vi "Logging Message Loop.vi"(8 "error in (no error)":cluster{"状态":bool, "代码":i32, "源":string} caption="错误输入（无错误）", 10 "数据队列":refnum<queue>, 11 "消息队列":T1) -> (0 "error out":cluster{"状态":bool, "代码":i32, "源":string} caption="错误输出")   [LabVIEW 2015, in "DAQ.lvlib"]
doc: "消息循环子VI负责处理与记录数据相关的消息。"
uses:
  DAQ.lvlib
  support/Message Queue/All Message Queues Sample Panel.ctl
  support/Message Queue/Message Cluster.ctl
  Support/Logging Configuration.ctl
  Support/Logging State.ctl
  support/Message Queue/Enqueue Message (Single).vi
  <vilib>/Utility/error.llb/Error Cluster From Error Code.vi
  <vilib>/ErrorRing/Error Ring.xnode
  support/Message Queue/Message Queue.lvlib
  Utility VIs/Utility VIs.lvlib
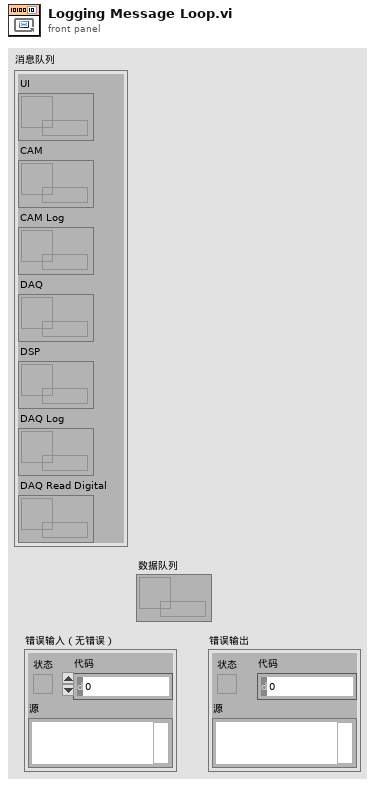
[diagram p1: front panel]
types:
  T1 = typedef "Message Queue.lvlib/All Message Queues Sample Panel.ctl" = cluster{"UI":refnum<queue>, "CAM":refnum<queue>, "CAM Log":refnum<queue>, "DAQ":refnum<queue>, "DSP":refnum<queue>, "DAQ Log":refnum<queue>, "DAQ Read Digital":refnum<queue>}
  T2 = typedef "DAQ.lvlib/Logging State.ctl" = enum16{"Idle", "Logging"}
  T3 = typedef "DAQ.lvlib/Logging Configuration.ctl" = cluster{"记录文件基路径":path}
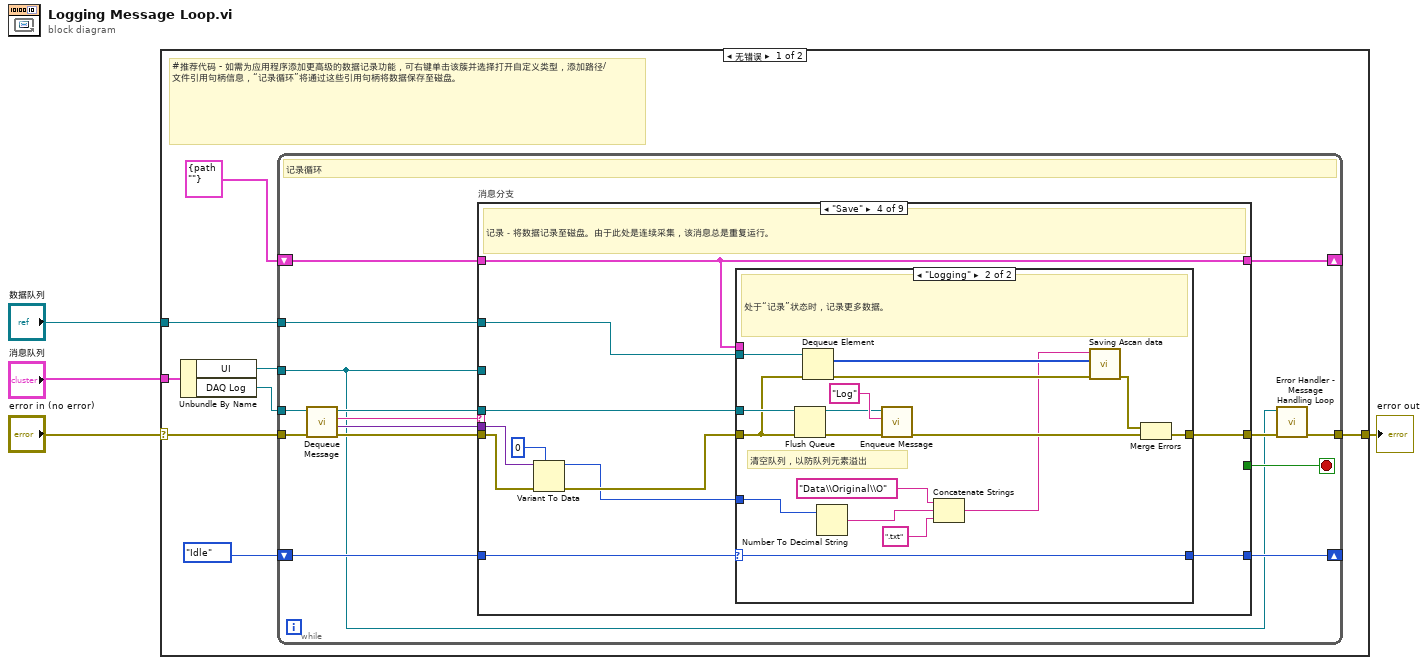
[diagram p0: block diagram]
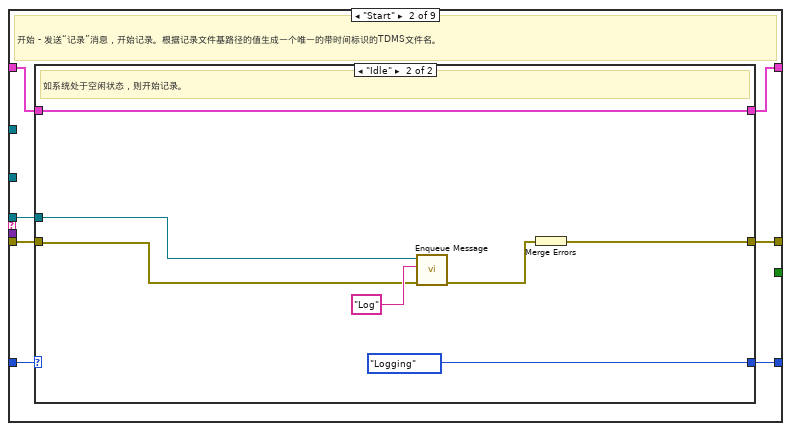
[diagram p3: hidden frame]
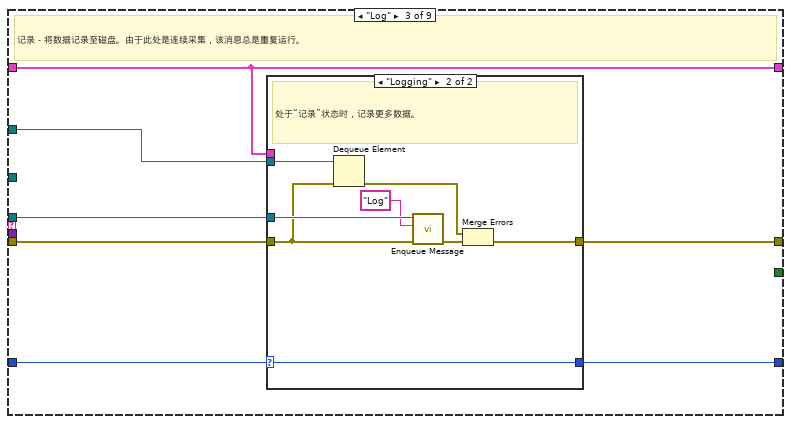
[diagram p5: hidden frame]
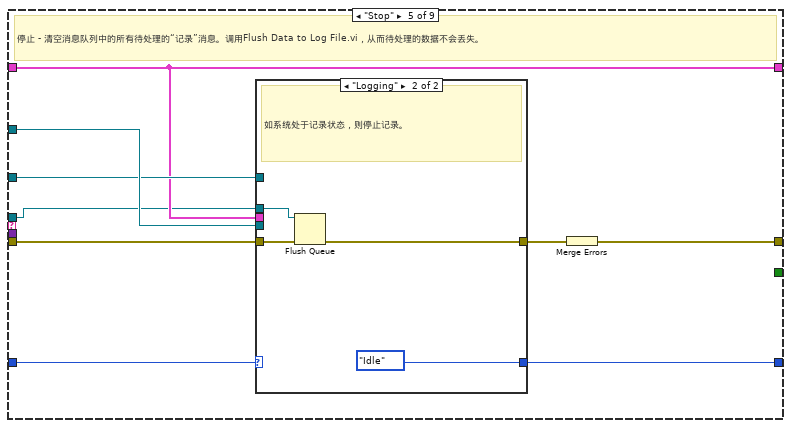
[diagram p8: hidden frame]
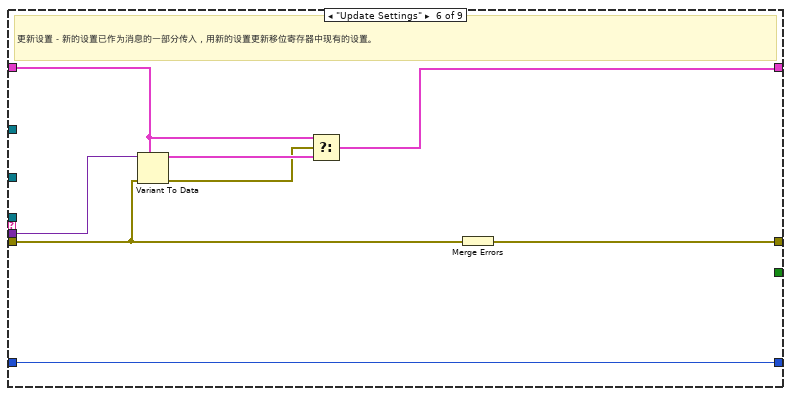
[diagram p10: hidden frame]
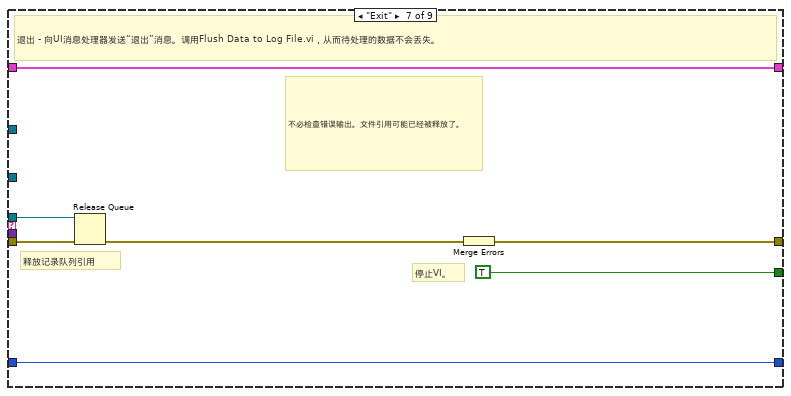
[diagram p11: hidden frame]
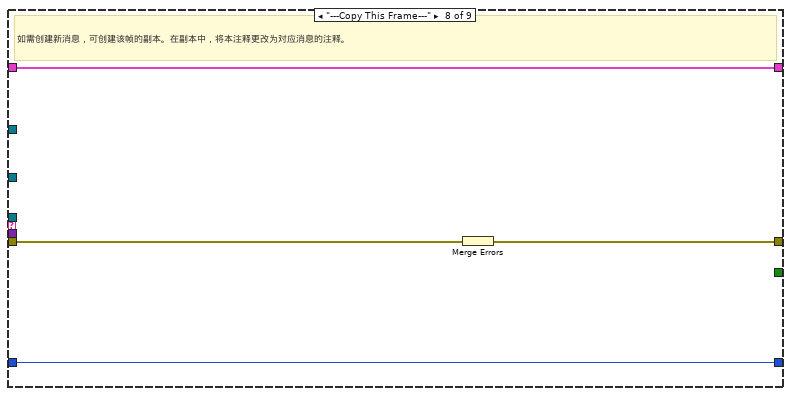
[diagram p12: hidden frame]
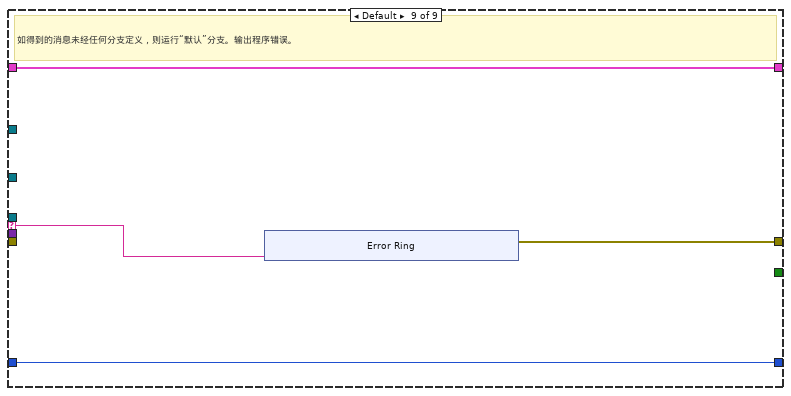
[diagram p13: hidden frame]
diagram:
  n1 = case shown="无错误" "error in (no error)" {
    selector: "error in (no error)" -> [w9 w140]
    tunnel: "消息队列" -> [w12 _]
    tunnel: [w10 w140] -> w4
    tunnel: "数据队列" -> [w8 _]
    frame No Error {
      # "#推荐代码 - 如需为应用程序添加更高级的数据记录功能，可右键单击该簇并选择打开自定义类型，添加路径/文件引用句柄信息，“记录循环”将通过这些引用句柄将数据保存至磁盘。"
      n2 = Unbundle By Name(w12) -> ("UI"=w7:refnum<queue>, "DAQ Log"=w11:refnum<queue>)
      n3 = while {
        tunnel: w11 -> [w19]
        shift-right: [w26] -> _
        shift-left: T3 {"记录文件基路径"=path ""} ("记录配置") -> [w27]
        tunnel: w7 -> [w13]
        tunnel: w8 -> [w18]
        shift-right: [w16] -> _
        shift-left: Logging_State."Idle" ("记录状态") -> [w17]
        tunnel: w9 -> [w24]
        tunnel: [w15] -> w10
        stop <- w25 stop-if-true
        # "记录循环"
        n4 = call "Dequeue Message.vi"("error in (no error)"=w24, "消息队列"=w19) -> ("error out"=w23:cluster{"状态":bool, "代码":i32, "源":string}, "消息数据"=w21:variant, "消息"=w22:string, "消息队列副本"=w20:refnum<queue>)  [unwired: 6 in]
        n5 = case "消息分支" shown="\"Save\"" w22 {
          selector: w22 -> [_ _ _ _ _ _ _ _ w129]
          tunnel: w20 -> [_ w36 w53 w74 w95 _ w121 _ _]
          tunnel: w23 -> [w29 w35 w51 w67 w100 w111 w122 w128 _]
          tunnel: [w29 w37 w54 w75 w103 w117 w123 w126 w130] -> w14
          tunnel: w27 -> [w30 w34 w50 w72 w96 w115 w119 w127 w132]
          tunnel: [w30 w33 w50 w72 w96 w112 w119 w127 w132] -> w26
          tunnel: [_ _ _ _ _ _ TRUE _ _] -> w25
          tunnel: w21 -> [_ _ _ w69 _ w116 _ _ _]
          tunnel: w13 -> [_ _ _ _ w97 _ _ _ _]
          tunnel: w18 -> [_ _ w52 w73 w101 _ _ _ _]
          tunnel: w17 -> [w28 w32 w49 w71 w99 w110 w118 w125 w131]
          tunnel: [w28 w31 w48 w70 w98 w110 w118 w125 w131] -> w16
          frame "Initialize" {
            # "初始化－第一次启动时将被调用。当前不包含任何操作。"
          }
          frame "Start" {
            # "开始 - 发送“记录”消息，开始记录。根据记录文件基路径的值生成一个唯一的带时间标识的TDMS文件名。"
            n6 = case shown="\"Idle\"" w32 {
              selector: w32 -> [w39 _]
              tunnel: [w38 w44] -> w37
              tunnel: w36 -> [_ w45]
              tunnel: w35 -> [w38 w43]
              tunnel: w34 -> [w40 w41]
              tunnel: [w40 w41] -> w33
              tunnel: [w39 Logging_State."Logging" ("记录状态")] -> w31
              frame "Logging" {
                # "系统已处于记录状态。忽略“开始”消息。"
              }
              frame "Idle" {
                # "如系统处于空闲状态，则开始记录。"
                n7 = call-poly "Enqueue Message.vi"("error in (no error)"=w43, "消息"="Log" ("Message"), "消息队列"=w45) -> ("error out"=w46:cluster{"状态":bool, "代码":i32, "源":string})  [unwired: 7 in, 1 out]
                n8 = Merge Errors(w46) -> (w44:errorcluster)
              }
            }
          }
          frame "Log" {
            # "记录－将数据记录至磁盘。由于此处是连续采集，该消息总是重复运行。"
            n9 = case shown="\"Logging\"" w49 {
              selector: w49 -> [w56 w60]
              tunnel: [w55 w64] -> w54
              tunnel: w53 -> [_ w62]
              tunnel: w52 -> [_ w59]
              tunnel: w51 -> [w55 w58]
              tunnel: w50 -> [_ _]
              tunnel: [w56 w60] -> w48
              frame "Idle" {
                # "如记录处于空闲状态，则忽略“记录”消息。"
              }
              frame "Logging" {
                # "处于“记录”状态时，记录更多数据。"
                n10 = Dequeue Element(queue=w59, error in (no error)=w58) -> (error out=w57:errorcluster)  [unwired: 1 in, 3 out]
                n11 = call-poly "Enqueue Message.vi"("error in (no error)"=w58, "消息"="Log" ("Message"), "消息队列"=w62) -> ("error out"=w63:cluster{"状态":bool, "代码":i32, "源":string})  [unwired: 7 in, 1 out]
                n12 = Merge Errors(w57, w63) -> (w64:errorcluster)
              }
            }
          }
          frame "Save" {
            # "记录－将数据记录至磁盘。由于此处是连续采集，该消息总是重复运行。"
            n13 = Variant To Data(error in=w67, type=0, Variant=w69) -> (data=w65:i32, error out=w66:errorcluster)
            n14 = case shown="\"Logging\"" w71 {
              selector: w71 -> [w77 w91]
              tunnel: [w76 w94] -> w75
              tunnel: w74 -> [_ w89]
              tunnel: w73 -> [_ w90]
              tunnel: w66 -> [w76 w87]
              tunnel: w72 -> [_ _]
              tunnel: [w77 w91] -> w70
              tunnel: w65 -> [_ w79]
              frame "Idle" {
                # "如记录处于空闲状态，则忽略“记录”消息。"
              }
              frame "Logging" {
                # "清空队列，以防队列元素溢出"
                # "处于“记录”状态时，记录更多数据。"
                n15 = Flush Queue(queue=w89, error in (no error)=w87) -> (queue out=w88:refnum<queue>, error out=w86:errorcluster)  [unwired: 1 out]
                n16 = Dequeue Element(queue=w90, error in (no error)=w87) -> (element=w85:i16[], error out=w84:errorcluster)  [unwired: 1 in, 2 out]
                n17 = Number To Decimal String(number=w79) -> (decimal integer string=w81:string)  [unwired: 1 in]
                n18 = call-poly "Enqueue Message.vi"("error in (no error)"=w86, "消息"="Log" ("Message"), "消息队列"=w88) -> ("error out"=w93:cluster{"状态":bool, "代码":i32, "源":string})  [unwired: 7 in, 1 out]
                n19 = Concatenate Strings("Data\\Original\\O", w81, ".txt" ("字符串")) -> (w78:string)
                n20 = call "Saving Ascan data.vi"("error in (no error)"=w84, "Ascan Data"=w85, "名称或相对路径"=w78) -> ("error out"=w83:errorcluster)  [unwired: 8 in]
                n21 = Merge Errors(w83, w93) -> (w94:errorcluster)
              }
            }
          }
          frame "Stop" {
            # "停止 - 清空消息队列中的所有待处理的“记录”消息。调用Flush Data to Log File.vi，从而待处理的数据不会丢失。"
            n22 = case shown="\"Logging\"" w99 {
              selector: w99 -> [w104 _]
              tunnel: [w105 w106] -> w102
              tunnel: w101 -> [_ _]
              tunnel: w96 -> [_ _]
              tunnel: w100 -> [w105 w108]
              tunnel: [w104 Logging_State."Idle" ("记录状态")] -> w98
              tunnel: w97 -> [_ _]
              tunnel: w95 -> [_ w107]
              frame "Idle" {
                # "系统已处于空闲状态。忽略“停止”消息。"
              }
              frame "Logging" {
                # "如系统处于记录状态，则停止记录。"
                n23 = Flush Queue(queue=w107, error in (no error)=w108) -> (error out=w106:errorcluster)  [unwired: 2 out]
              }
            }
            n24 = Merge Errors(w102) -> (w103:errorcluster)
          }
          frame "Update Settings" {
            # "更新设置－新的设置已作为消息的一部分传入，用新的设置更新移位寄存器中现有的设置。"
            n25 = Variant To Data(error in=w111, type=w115, Variant=w116) -> (data=w114:T3, error out=w113:errorcluster)
            n26 = Select(t=w115, s=w113, f=w114) -> (s? t:f=w112:T3)
            n27 = Merge Errors(w111) -> (w117:errorcluster)
          }
          frame "Exit" {
            # "不必检查错误输出。文件引用可能已经被释放了。"
            # "释放记录队列引用"
            # "停止VI。"
            # "退出 - 向UI消息处理器发送“退出”消息。调用Flush Data to Log File.vi，从而待处理的数据不会丢失。"
            n28 = Release Queue(queue=w121, error in (no error)=w122) -> (error out=w120:errorcluster)  [unwired: 1 in, 2 out]
            n29 = Merge Errors(w120) -> (w123:errorcluster)
          }
          frame "---Copy This Frame---" {
            # "如需创建新消息，可创建该帧的副本。在副本中，将本注释更改为对应消息的注释。"
            n30 = Merge Errors(w128) -> (w126:errorcluster)
          }
          frame Default {
            # "如得到的消息未经任何分支定义，则运行“默认”分支。输出程序错误。"
            n31 = xnode ("Error Ring")("参数 0"=w129) -> ("错误输出"=w130:errorcluster)
          }
        }
        n32 = call "Error Handler - Message Handling Loop.vi"("error in (no error)"=w14, "消息队列"=w13) -> ("错误输入副本"=w15:cluster{"状态":bool, "代码":i32, "源":string})  [unwired: 8 in, 1 out]
      }
    }
    frame Error {
    }
  }
  "error out" <- w4
